vi "Set Panes to Origins.vi"(8 "error in (no error)":errorcluster, 11 "IViewable In":refnum<class "IViewable.lvclass">) -> (0 "error out":errorcluster, 3 "IViewable Out":refnum<class "IViewable.lvclass">)   [LabVIEW 2015, in "IViewable.lvlib" / "IViewable.lvclass"]
doc: "<License>\nCopyright © 2017 Composed Systems, LLC | All rights reserved\nwww.composed.io\n\nAuthor: Ethan Stern <ethan.stern@composed.io>\n\nThis software is provided \"AS IS\" WITHOUT WARRANTIES, either express or implied, AND IS FOR EDUCATIONAL PURPOSES ONLY.\n</License>"
uses:
  IViewable.lvclass
  <vilib>/Utility/miscctls.llb/LVPointTypeDef.ctl
  IViewable.lvclass/IViewable.ctl
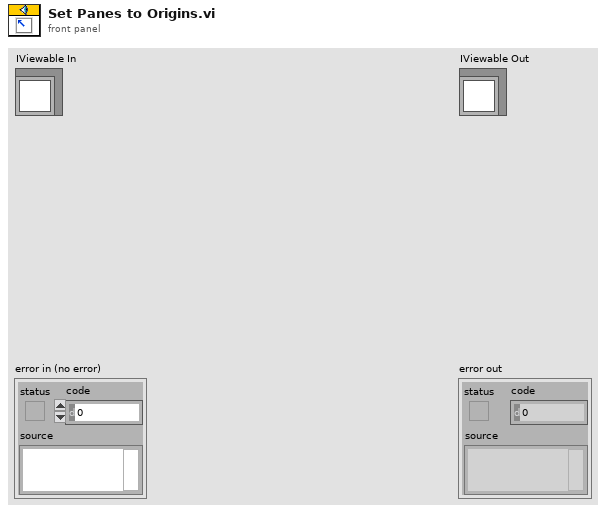
[diagram p1: front panel]
types:
  T1 = typedef "LVPointTypeDef.ctl" = cluster{"Horizontal":i16, "Vertical":i16}
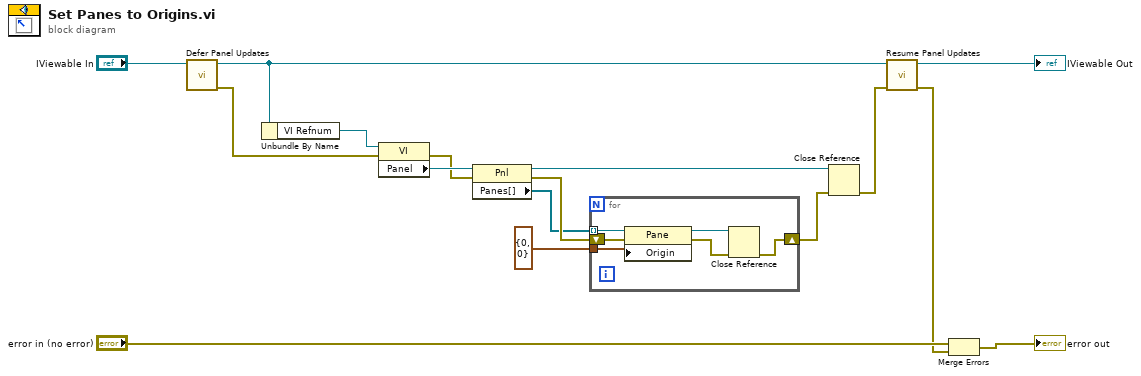
[diagram p0: block diagram]
diagram:
  n1 = call-dynamic "Defer Panel Updates.vi"("IViewable In"="IViewable In") -> ("error out"=w1:errorcluster, "IViewable Out"=w2:refnum<class "IViewable.lvclass">)  [unwired: 9 in]
  n2 = Unbundle By Name(w2) -> ("VI Refnum"=w12:refnum<vi>)
  n3 = property class="VI"(reference=w12, error in=w1) -> (error out=w10:errorcluster, "Panel"=w11:refnum<vi>)  [unwired: 1 out]
  n4 = property class="Pnl"(reference=w11, error in=w10) -> (reference out=w9:refnum<vi>, error out=w8:errorcluster, "Panes[]"=w6:refnum<vi>[])
  n5 = for {
    tunnel: w6 -> [w22] mode=indexing
    shift-right: [w17] -> w5
    shift-left: w8 -> [w21]
    tunnel: T1 {"Horizontal"=0, "Vertical"=0} ("Origin") -> [w20]
    n6 = property class="Pane"(reference=w22, error in=w21, "Origin"=w20) -> (reference out=w19:refnum<vi>, error out=w18:errorcluster)
    n7 = Close Reference(reference=w19, error in (no error)=w18) -> (error out=w17:errorcluster)
  }
  n8 = Close Reference(reference=w9, error in (no error)=w5) -> (error out=w4:errorcluster)
  n9 = call-dynamic "Resume Panel Updates.vi"("error in (no error)"=w4, "IViewable In"=w2) -> ("error out"=w3:errorcluster, "IViewable Out"=→"IViewable Out":refnum<class "IViewable.lvclass">)  [unwired: 8 in]
  n10 = Merge Errors("error in (no error)", w3) -> (→"error out":errorcluster)
